vi "例5.10  “解除捆绑”函数.vi"() -> ()   [LabVIEW 2017]
panel:
  out "布尔":bool
  out "数值":i32
  out "字符串":string
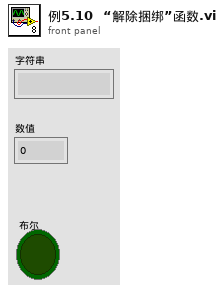
[diagram p1: front panel]
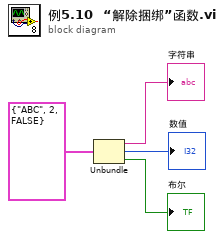
[diagram p0: block diagram]
diagram:
  n1 = Unbundle(cluster{string, i32, bool} {"ABC", 2, FALSE}) -> (→"字符串":string, →"数值":i32, →"布尔":bool)
